vi "Write UUT Data.vi"(8 "error in (no error)":errorcluster, 10 "UUT Data (\"*IDN?\\r\\n\")":string="\"*IDN?\r\n\"", 11 "VISA resource name":refnum<visa-resource-name>) -> (0 "error out":errorcluster, 3 "VISA resource name out":refnum<visa-resource-name>)   [LabVIEW 2014, in "Fluke 5XXX Series Multicalibrators.lvlib"]
doc: "This VI sends data to the UUT serial port in binary block or string data format over the Calibrator rear panel SERIAL 2 TO UUT serial port. The command may be sent over gpib or RS-232 ports, but applies to SERIAL 2 TO UUT serial port operation. Include a line feed (RS-232) character to terminate the block data or End or Identify (EOI) command (IEEE-488).\n\nNote:\n\nThis VI is available only for instrument models 5500A and 5520A."
uses:
  Fluke 5XXX Series Multicalibrators.lvlib
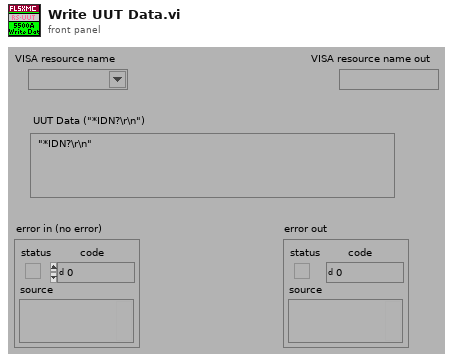
[diagram p1: front panel]
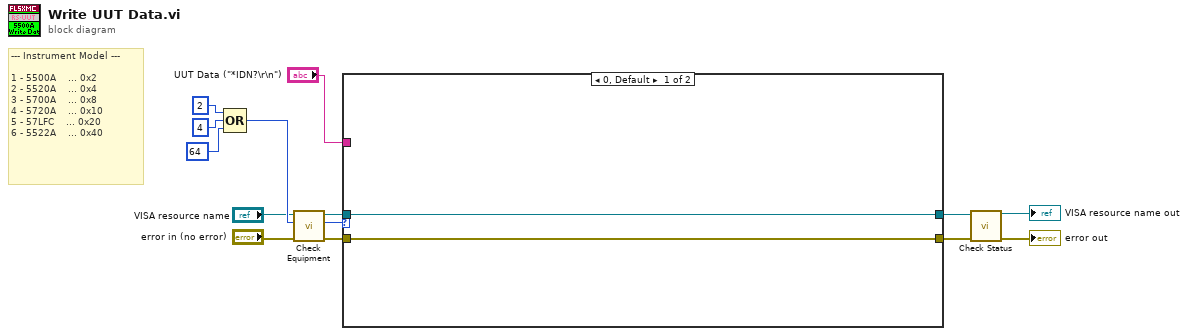
[diagram p0: block diagram]
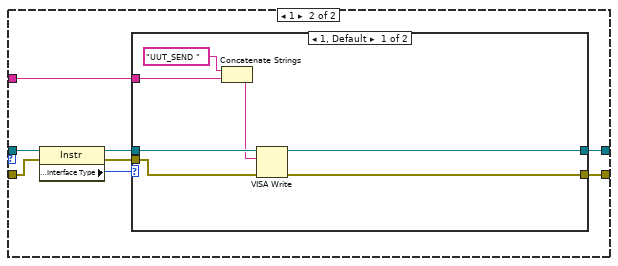
[diagram p2: hidden frame]
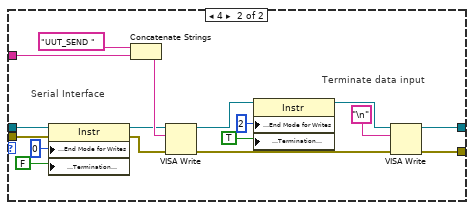
[diagram p3: hidden frame]
diagram:
  # "--- Instrument Model ---\n\n1 - 5500A    ... 0x2\n2 - 5520A    ... 0x4\n3 - 5700A    ... 0x8\n4 - 5720A    ... 0x10\n5 - 57LFC    ... 0x20\n6 - 5522A    ... 0x40"
  n1 = Compound Arithmetic op=OR(u32 2, u32 4, 64 ("Numeric")) -> (w12:u32)
  n2 = call "Check Equipment.vi"("error in (no error)"="error in (no error)", "Bit Mask"=w12, "VISA resource name"="VISA resource name") -> ("error out"=w14:errorcluster, "Present?"=w9:u32, "VISA resource name out"=w13:refnum<visa-resource-name>)  [unwired: 6 in]
  n3 = case shown="0, Default" w9 {
    tunnel: w14 -> [w15 w17]
    tunnel: w13 -> [w16 w18]
    tunnel: [w16 w20] -> w2
    tunnel: [w15 w19] -> w5
    tunnel: "UUT Data (\"*IDN?\\r\\n\")" -> [_ w21]
    frame 0, Default {
    }
    frame 1 {
      n4 = property class="Instr"(reference=w18, error in=w17) -> (reference out=w23:refnum<visa-resource-name>, error out=w22:errorcluster, "Interface Information:Interface Type"=w24:u16)
      n5 = case shown="1, Default" w24 {
        tunnel: w23 -> [w31 w44]
        tunnel: w22 -> [w29 w43]
        tunnel: w21 -> [w27 w38]
        tunnel: [w30 w36] -> w20
        tunnel: [w28 w35] -> w19
        frame 1, Default {
          n6 = Concatenate Strings("UUT_SEND " ("Substring"), w27) -> (w26:string)
          n7 = VISA Write(VISA resource name=w31, write buffer=w26, error in (no error)=w29) -> (VISA resource name out=w30:refnum<visa-resource-name>, error out=w28:errorcluster)  [unwired: 1 out]
        }
        frame 4 {
          # "Terminate data input"
          # "Serial Interface"
          n8 = property class="Instr"(reference=w44, error in=w43, "Serial Settings:End Mode for Writes"=u16 0 ("ASRL End In"), "Message Based Settings:Termination Character Enable"=FALSE ("TermChar En")) -> (reference out=w39:refnum<visa-resource-name>, error out=w40:errorcluster)
          n9 = Concatenate Strings("UUT_SEND " ("Substring"), w38) -> (w42:string)
          n10 = VISA Write(VISA resource name=w39, write buffer=w42, error in (no error)=w40) -> (VISA resource name out=w37:refnum<visa-resource-name>, error out=w33:errorcluster)  [unwired: 1 out]
          n11 = property class="Instr"(reference=w37, "Serial Settings:End Mode for Writes"=u16 2 ("ASRL End In"), "Message Based Settings:Termination Character Enable"=TRUE ("TermChar En")) -> (reference out=w34:refnum<visa-resource-name>)  [unwired: 1 in, 1 out]
          n12 = VISA Write(VISA resource name=w34, write buffer="\n" ("write buffer (\"\")"), error in (no error)=w33) -> (VISA resource name out=w36:refnum<visa-resource-name>, error out=w35:errorcluster)  [unwired: 1 out]
        }
      }
    }
  }
  n13 = call "Check Status.vi"("VISA resource name"=w2, "error in (no error)"=w5) -> ("VISA resource name out"=→"VISA resource name out":refnum<visa-resource-name>, "error out"=→"error out":errorcluster)  [unwired: 12 in]
